vi "Init Model(SubVI).vi"() -> (2 "Scene:New Object":refnum<vi>, 3 "SceneObject out":refnum<vi>)   [LabVIEW 2018]
uses:
  <vilib>/picture/3D Picture Control/Object/Create Object (name).vi
  <vilib>/picture/3D Picture Control/NI_3D Picture Control.lvlib
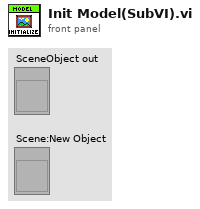
[diagram p1: front panel]
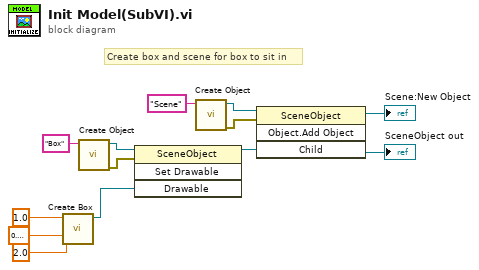
[diagram p0: block diagram]
diagram:
  # "Create box and scene for box to sit in"
  n1 = call <vilib>:"Create Box.vi"("Length Z"=sgl 2.0, "Length Y"=sgl 0.2, "Length X"=sgl 1.0) -> ("New Box Refnum"=w6:refnum<vi>)  [unwired: 7 in, 1 out]
  n2 = call-poly <vilib>:"Create Object.vi"("Name"="Box") -> ("error out"=w5:errorcluster, "Scene:New Object"=w3:refnum<vi>)  [unwired: 9 in]
  n3 = invoke class="SceneObject" method="Set Drawable"(reference=w3, error in=w5, "Drawable"=w6) -> (reference out=w13:refnum<vi>)  [unwired: 1 in, 3 out]
  n4 = call-poly <vilib>:"Create Object.vi"("Name"="Scene") -> ("error out"=w12:errorcluster, "Scene:New Object"=w11:refnum<vi>)  [unwired: 9 in]
  n5 = invoke class="SceneObject" method="Object.Add Object"(reference=w11, error in=w12, "Child"=w13) -> (reference out=→"Scene:New Object":refnum<vi>, "Child"=→"SceneObject out":refnum<vi>)  [unwired: 1 in, 2 out]
